vi "PFI-28000-Utils_Parse String Value.vi"(0 "String":string, 11 "error in (no error)":errorcluster) -> (4 "String Value":string, 6 "Channels":i32[](array[numeric]), 15 "error out":errorcluster)   [LabVIEW 2017, in "PFI-28000-Utils.lvlib"]
uses:
  PFI-28000-Utils.lvlib
  <vilib>/regexp/Match Regular Expression.xnode
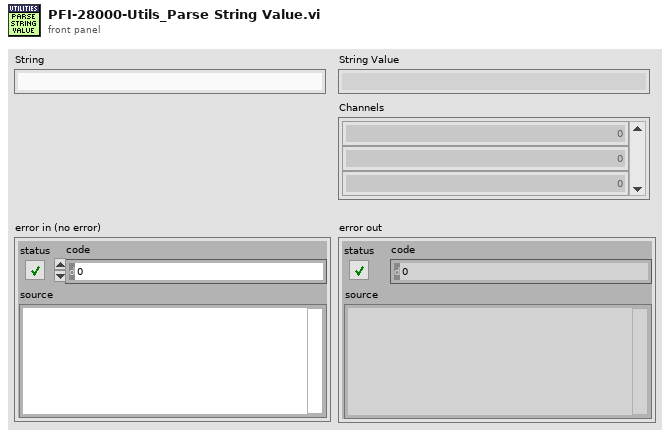
[diagram p1: front panel]
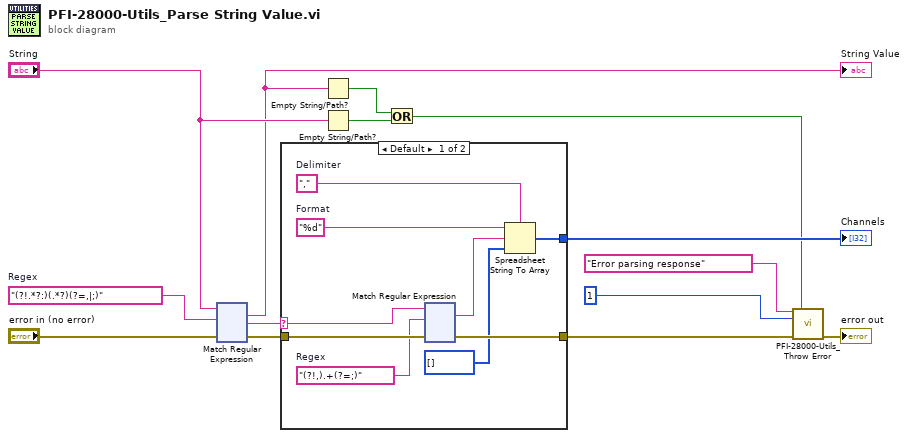
[diagram p0: block diagram]
diagram:
  w14 = "(?!.*?:)(.*?)(?=,|;)"  # Regex
  n1 = xnode "Match Regular Expression"("input string"="String", "regular expression"=w14, "error in"="error in (no error)") -> ("whole match"=w4:string, "after match"=w11:string, "error out"=w12:errorcluster)  [unwired: 3 in, 2 out]
  "String Value" <- w4
  n2 = case shown="Default" w11 {
    selector: w11 -> [w16 _]
    tunnel: w12 -> [w23 w138]
    tunnel: [w22 w138] -> w9
    tunnel: [w18 _] -> w10
    frame Default {
      w19 = ","  # Delimiter
      w20 = "%d"  # Format
      w17 = "(?!,).+(?=;)"  # Regex
      n3 = xnode "Match Regular Expression"("input string"=w16, "regular expression"=w17, "error in"=w23) -> ("whole match"=w15:string, "error out"=w22:errorcluster)  [unwired: 3 in, 3 out]
      n4 = Spreadsheet String To Array(delimiter (Tab)=w19, format string=w20, spreadsheet string=w15, array type (2D Dbl)=i32[] [] ("Channels")) -> (array=w18:i32[])
    }
    frame ";" {
    }
  }
  "Channels" <- w10
  n5 = Empty String/Path?(string/path=w4) -> (empty?=w3:bool)
  n6 = Empty String/Path?(string/path="String") -> (empty?=w2:bool)
  n7 = Or(x=w3, y=w2) -> (x .or. y?=w1:bool)
  n8 = call "PFI-28000-Utils_Throw Error.vi"("Error Message"="Error parsing response" ("empty string"), "Throw?"=w1, "Error Code"=1, "error in (no error)"=w9) -> ("error out"=→"error out":errorcluster)  [unwired: 11 in]
